vi "CrossTurn Motor Controller.vi"(8 "Speed":dbl(slide) scale=0.0..1.0, 9 "Right":bool, 10 "Left":bool, 11 "Forward":bool) -> (0 "Duty Cycle B2":dbl, 1 "Duty Cycle B1":dbl, 2 "Duty Cycle A2":dbl, 3 "Duty Cycle A1":dbl)   [LabVIEW 2019]
doc: "The motor controlling programmation for the Automatic Drive.\nInputs Forward, Left, Right are booleans to indicate in which direction you would like to drive.\nInput Speed is to limit the speed at which the motors will turn."
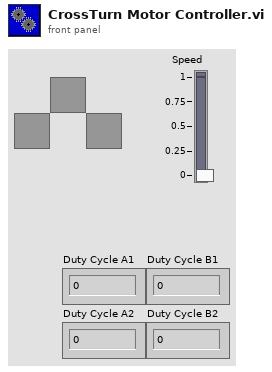
[diagram p1: front panel]
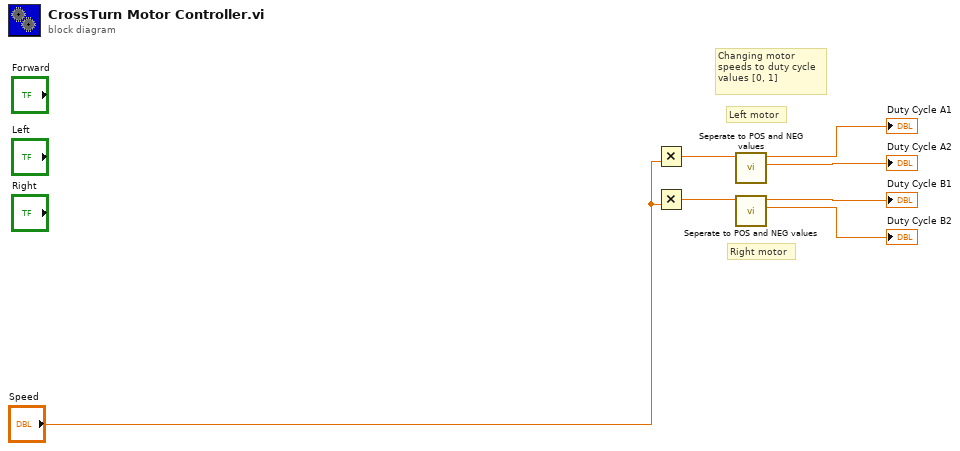
[diagram p0: block diagram]
diagram:
  # "Changing motor\nspeeds to duty cycle\nvalues [0, 1]"
  # "Right motor"
  # "Left motor"
  n1 = Multiply(y="Speed") -> (x*y=w6:dbl)  [unwired: 1 in]
  n2 = Multiply(y="Speed") -> (x*y=w5:dbl)  [unwired: 1 in]
  n3 = call "Seperate to POS and NEG values.vi"("Motorspeed"=w6) -> ("Duty Cycle 2"=→"Duty Cycle A2":dbl, "Duty Cycle 1"=→"Duty Cycle A1":dbl)  [unwired: 9 in]
  n4 = call "Seperate to POS and NEG values.vi"("Motorspeed"=w5) -> ("Duty Cycle 2"=→"Duty Cycle B2":dbl, "Duty Cycle 1"=→"Duty Cycle B1":dbl)  [unwired: 9 in]
